vi "Prevent Sleeping.vi"(8 "error in (no error)":errorcluster, 11 "keep screen on":bool=TRUE) -> (0 "error out":errorcluster)   [LabVIEW 2024, in "VIPM Power Requests.lvlib"]
doc: "Prevents computer from going to sleep and optionally keeps screen on."
uses:
  VIPM Power Requests.lvlib
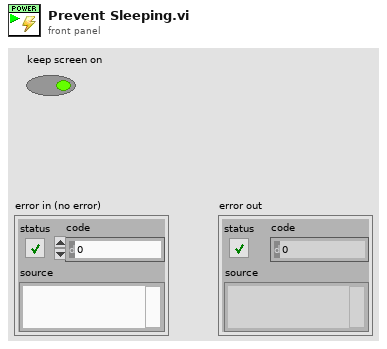
[diagram p1: front panel]
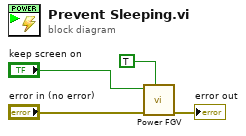
[diagram p0: block diagram]
diagram:
  n1 = call "Power FGV.vi"("prevent sleep"=TRUE, "error in (no error)"="error in (no error)", "keep screen on"="keep screen on") -> ("error out"=→"error out":errorcluster)  [unwired: 8 in]
